vi "Find Line.vi"(9 "Z":dbl, 10 "X":dbl, 11 "All Lines":T1) -> (0 "Distance to nearest":dbl, 1 "Index on Line":i32, 2 "Nearest Line":i32, 3 "Line found?":bool)   [LabVIEW 2014, in "Map Data.lvlib"]
uses:
  Map Data.lvlib
  All-Lines.ctl
  LineCluster.ctl
  LineConnection.ctl
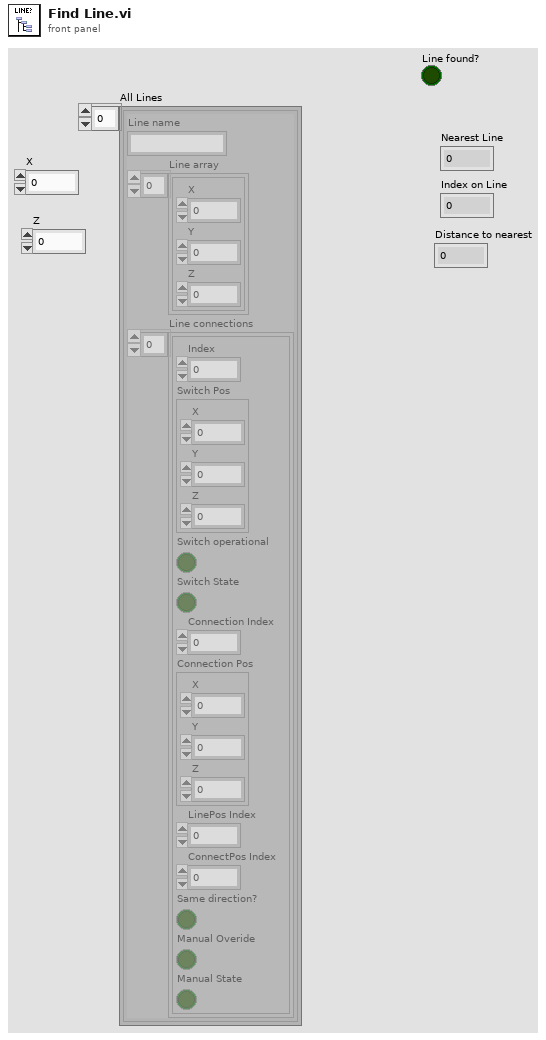
[diagram p1: front panel]
types:
  T1 = typedef "Map Data.lvlib/All-Lines.ctl" = T2[]
  T2 = typedef "Map Data.lvlib/LineCluster.ctl" = cluster{"Line name":string, "Line array":cluster{"X":dbl, "Y":dbl, "Z":dbl}[], "Line connections":T3[]}
  T3 = typedef "LineConnection.ctl" = cluster{"Index":i32, "Switch Pos":cluster{"X":dbl, "Y":dbl, "Z":dbl}, "Switch operational":bool, "Switch State":bool, "Connection Index":i32, "Connection Pos":cluster{"X":dbl, "Y":dbl, "Z":dbl}, "LinePos Index":i32, "ConnectPos Index":i32, "Same direction?":bool, "Manual Overide":bool, "Manual State":bool}
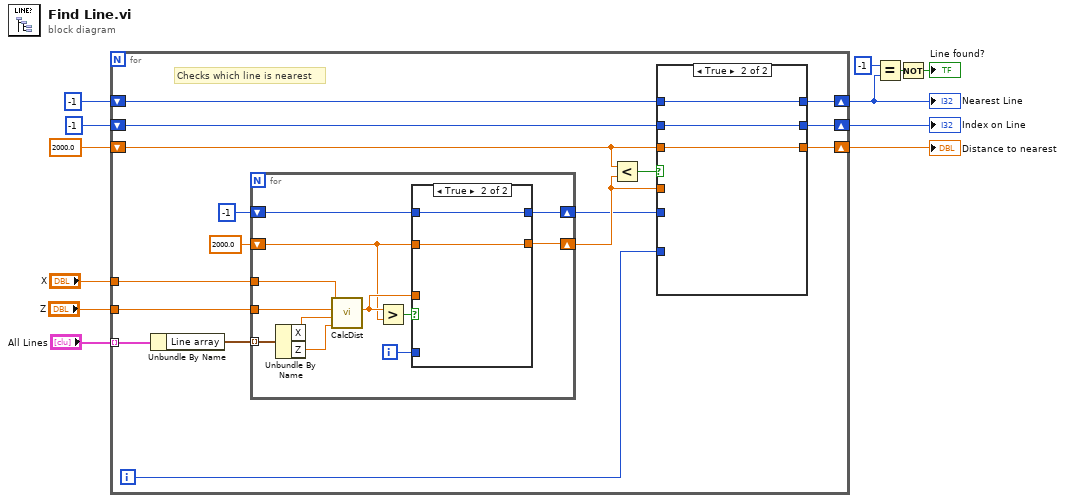
[diagram p0: block diagram]
diagram:
  n1 = for {
    tunnel: "All Lines" -> [w28] mode=indexing
    tunnel: "X" -> [w26]
    tunnel: "Z" -> [w25]
    shift-right: [w23] -> w10
    shift-left: 2000.0 ("Distance") -> [w19]
    shift-right: [w21] -> w6
    shift-left: -1 -> [w20]
    shift-right: [w13] -> w1
    shift-left: -1 -> [w16]
    i -> [w22]
    # "Checks which line is nearest"
    n2 = Unbundle By Name(w28) -> ("Line array"=w27:cluster{"X":dbl, "Y":dbl, "Z":dbl}[])
    n3 = for {
      tunnel: w26 -> [w46]
      tunnel: w27 -> [w45] mode=indexing
      tunnel: w25 -> [w41]
      shift-right: [w38] -> w18
      shift-left: 2000.0 ("Distance") -> [w39]
      shift-right: [w35] -> w14
      shift-left: -1 -> [w37]
      i -> [w36]
      n4 = Unbundle By Name(w45) -> ("X"=w42:dbl, "Z"=w43:dbl)
      n5 = call "CalcDist.vi"("Y2"=w43, "X2"=w42, "Y1"=w41, "X1"=w46) -> ("Distance"=w40:dbl)  [unwired: 7 in]
      n6 = Greater?(x=w40, y=w39) -> (0:w44:bool)
      n7 = case shown="True" w44 {
        tunnel: w40 -> [w48 _]
        tunnel: [w48 w50] -> w38
        tunnel: w39 -> [_ w50]
        tunnel: w37 -> [_ w49]
        tunnel: w36 -> [w47 _]
        tunnel: [w47 w49] -> w35
        frame False {
        }
        frame True {
        }
      }
    }
    n8 = Less?(x=w19, y=w18) -> (x < y?=w17:bool)
    n9 = case shown="True" w17 {
      tunnel: w18 -> [w31 _]
      tunnel: [w31 w33] -> w23
      tunnel: w19 -> [_ w33]
      tunnel: w22 -> [w30 _]
      tunnel: [w30 w34] -> w21
      tunnel: w20 -> [_ w34]
      tunnel: w16 -> [_ w32]
      tunnel: w14 -> [w29 _]
      tunnel: [w29 w32] -> w13
      frame False {
      }
      frame True {
      }
    }
  }
  "Nearest Line" <- w6
  "Distance to nearest" <- w10
  "Index on Line" <- w1
  n10 = Equal?(x=-1, y=w6) -> (x = y?=w4:bool)
  n11 = Not(x=w4) -> (.not. x?=→"Line found?":bool)
